vi "Stop Output Panel.vi"(8 "error in (no error)":errorcluster, 9 "Panel Host":refnum<vi>, 10 "Panel VI in":refnum<vi>, 11 "CallEXEStep in":refnum<class "CallEXEStep.lvclass">) -> (0 "error out":errorcluster, 3 "CallEXEStep out":refnum<class "CallEXEStep.lvclass">)   [LabVIEW 2015, in "CallEXEStep.lvclass"]
uses:
  CallEXEStep.lvclass
  Step.lvclass
  Project.lvclass
  Editor/Editor.lvclass
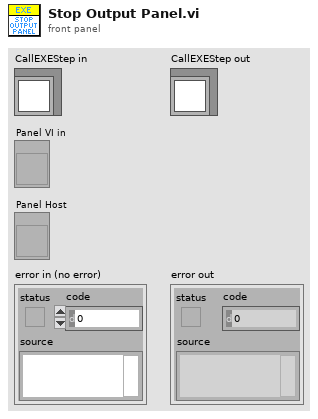
[diagram p1: front panel]
types:
  T1 = typedef "Step.lvclass/STEP_OUTPUT.ctl" = cluster{"Label":string, "Name":string, "Data Type":T2, "Check Type":T3, "String Limit":string, "Lower Limit":dbl, "Upper Limit":dbl, "Boolean Limit":bool, "Ignore Case":bool, "Variable Name 1":string, "Limit Value Type 1":T4, "Variable Name 2":string, "Limit Value Type 2":T4}
  T2 = typedef "Step.lvclass/OUTPUT_DATA_TYPE.ctl" = enum16{"Boolean", "String", "Numeric", "Other"}
  T3 = typedef "Step.lvclass/OUTPUT_CHECK_TYPE.ctl" = enum16{"INVALID", "DO_NOT_CHECK", "RECORD", "VARIABLE", "EQUAL", "NOT_EQUAL", "STR_CONTAINS", "STR_START_WITH", "STR_END_WITH", "STR_REGEX_MATCH", "NUM_GT", "NUM_LT", "NUM_GE", "NUM_LE", "NUM_RANGE", "NUM_RANGE_BDY"}
  T4 = typedef "Step.lvclass/OUTPUT_VALUE_TYPE.ctl" = enum16{"Constant", "Variable"}
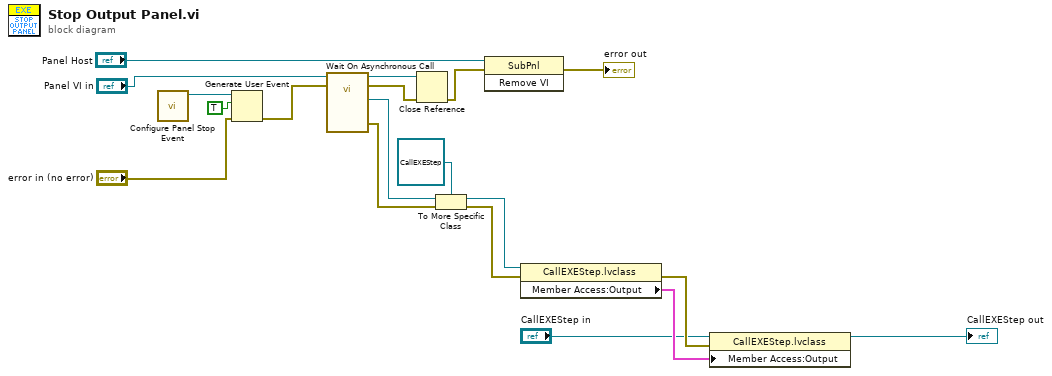
[diagram p0: block diagram]
diagram:
  n1 = call "Configure Panel Stop Event.vi"() -> ("Panel Stop event"=w15:refnum<user-event>)  [unwired: 11 in]
  n2 = Generate User Event(user event=w15, event data cluster=TRUE, error in="error in (no error)") -> (error out=w13:errorcluster)  [unwired: 1 in, 1 out]
  n3 = call-by-ref "Wait On Asynchronous Call"(reference="Panel VI in", error in=w13) -> (reference out=w19:refnum<vi>, error out=w18:errorcluster, 0:"error out"=w9:errorcluster, "Step out"=w8:refnum<class "Step.lvclass">)  [unwired: 10 in]
  n4 = Close Reference(reference=w19, error in (no error)=w18) -> (error out=w12:errorcluster)
  n5 = To More Specific Class(target class=refnum<class "CallEXEStep.lvclass"> refnum ("CallVIStep in"), reference=w8, error in=w9) -> (specific class reference=w5:refnum<class "CallEXEStep.lvclass">, error out=w6:errorcluster)
  n6 = invoke class="SubPnl" method="Remove VI"(reference="Panel Host", error in=w12) -> (error out=→"error out":errorcluster)  [unwired: 1 in, 2 out]
  n7 = property class="CallEXEStep.lvclass"(reference=w5, error in=w6) -> (error out=w3:errorcluster, "Member Access:Output"=w4:T1[])  [unwired: 1 out]
  n8 = property class="CallEXEStep.lvclass"(reference="CallEXEStep in", error in=w3, "Member Access:Output"=w4) -> (reference out=→"CallEXEStep out":refnum<class "CallEXEStep.lvclass">)  [unwired: 1 out]
